vi "Convert Array to IH.vi"(1 "Array":u8[](array[numeric])) -> (0 "IH":T1)   [LabVIEW 2013, in "VRI.lvlib"]
uses:
  VRI.lvlib
  _Type Defs/PhInt IH.ctl
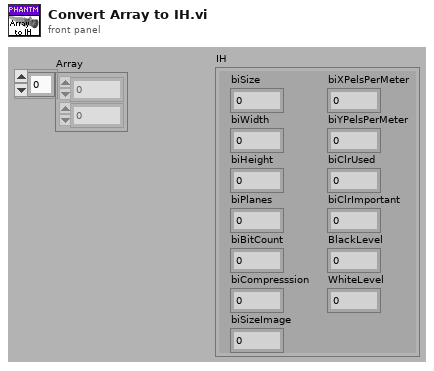
[diagram p1: front panel]
types:
  T1 = typedef "VRI.lvlib/PhInt IH.ctl" = cluster{"biSize":u32, "biWidth":i32, "biHeight":i32, "biPlanes":u16, "biBitCount":u16, "biCompresssion":u32, "biSizeImage":u32, "biXPelsPerMeter":i32, "biYPelsPerMeter":i32, "biClrUsed":u32, "biClrImportant":u32, "BlackLevel":i32, "WhiteLevel":i32}
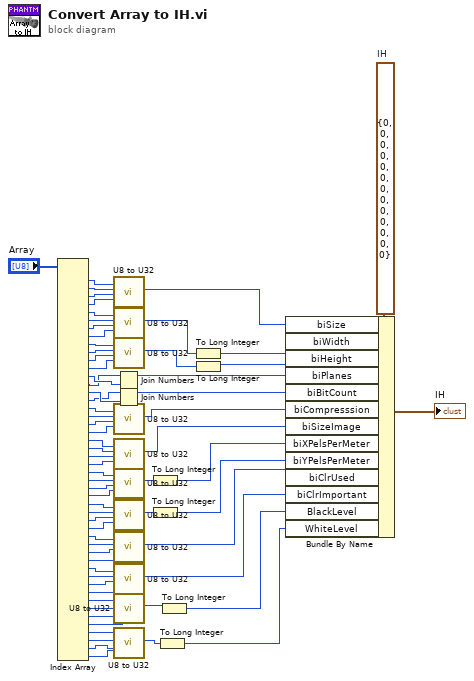
[diagram p0: block diagram]
diagram:
  w14 = T1 {"biSize"=0, "biWidth"=0, "biHeight"=0, "biPlanes"=0, "biBitCount"=0, "biCompresssion"=0, "biSizeImage"=0, "biXPelsPerMeter"=0, "biYPelsPerMeter"=0, "biClrUsed"=0, "biClrImportant"=0, "BlackLevel"=0, "WhiteLevel"=0}  # IH
  n1 = Index Array(array="Array") -> (element #1=w19:u8, element #2=w16:u8, element #3=w18:u8, element #4=w17:u8, element #5=w21:u8, element #6=w22:u8, element #7=w23:u8, element #8=w24:u8, element #9=w25:u8, element #10=w26:u8, element #11=w27:u8, element #12=w28:u8, element #13=w68:u8, element #14=w67:u8, element #15=w70:u8, element #16=w69:u8, element #17=w35:u8, element #18=w36:u8, element #19=w37:u8, element #20=w38:u8, element #21=w39:u8, element #22=w40:u8, element #23=w41:u8, element #24=w42:u8, element #25=w47:u8, element #26=w48:u8, element #27=w49:u8, element #28=w50:u8, element #29=w51:u8, element #30=w52:u8, element #31=w53:u8, element #32=w54:u8, element #33=w56:u8, element #34=w57:u8, element #35=w58:u8, element #36=w59:u8, element #37=w60:u8, element #38=w61:u8, element #39=w62:u8, element #40=w63:u8, element #41=w12:u8, element #42=w11:u8, element #43=w10:u8, element #44=w9:u8, element #45=w8:u8, element #46=w7:u8, element #47=w5:u8, element #48=w6:u8)  [unwired: 48 in]
  n2 = call "U8 to U32.vi"("Byte1"=w19, "Byte2"=w16, "Byte3"=w18, "Byte4"=w17) -> ("U32"=w20:u32)  [unwired: 1 in, 14 out]
  n3 = call "U8 to U32.vi"("Byte1"=w21, "Byte2"=w22, "Byte3"=w23, "Byte4"=w24) -> ("U32"=w29:u32)  [unwired: 1 in, 14 out]
  n4 = call "U8 to U32.vi"("Byte1"=w25, "Byte2"=w26, "Byte3"=w27, "Byte4"=w28) -> ("U32"=w30:u32)  [unwired: 1 in, 14 out]
  n5 = Join Numbers(hi=w67, lo=w68) -> ((hi.lo)=w33:u16)
  n6 = Join Numbers(hi=w69, lo=w70) -> ((hi.lo)=w34:u16)
  n7 = call "U8 to U32.vi"("Byte1"=w35, "Byte2"=w36, "Byte3"=w37, "Byte4"=w38) -> ("U32"=w43:u32)  [unwired: 1 in, 14 out]
  n8 = call "U8 to U32.vi"("Byte1"=w39, "Byte2"=w40, "Byte3"=w41, "Byte4"=w42) -> ("U32"=w44:u32)  [unwired: 1 in, 14 out]
  n9 = call "U8 to U32.vi"("Byte1"=w47, "Byte2"=w48, "Byte3"=w49, "Byte4"=w50) -> ("U32"=w46:u32)  [unwired: 1 in, 14 out]
  n10 = call "U8 to U32.vi"("Byte1"=w51, "Byte2"=w52, "Byte3"=w53, "Byte4"=w54) -> ("U32"=w45:u32)  [unwired: 1 in, 14 out]
  n11 = call "U8 to U32.vi"("Byte1"=w56, "Byte2"=w57, "Byte3"=w58, "Byte4"=w59) -> ("U32"=w64:u32)  [unwired: 1 in, 14 out]
  n12 = call "U8 to U32.vi"("Byte1"=w60, "Byte2"=w61, "Byte3"=w62, "Byte4"=w63) -> ("U32"=w65:u32)  [unwired: 1 in, 14 out]
  n13 = call "U8 to U32.vi"("Byte1"=w12, "Byte2"=w11, "Byte3"=w10, "Byte4"=w9) -> ("U32"=w4:u32)  [unwired: 1 in, 14 out]
  n14 = call "U8 to U32.vi"("Byte1"=w8, "Byte2"=w7, "Byte3"=w5, "Byte4"=w6) -> ("U32"=w2:u32)  [unwired: 1 in, 14 out]
  n15 = To Long Integer(number=w46) -> (32bit integer=w66:i32)
  n16 = To Long Integer(number=w45) -> (32bit integer=w55:i32)
  n17 = To Long Integer(number=w2) -> (32bit integer=w1:i32)
  n18 = To Long Integer(number=w4) -> (32bit integer=w3:i32)
  n19 = To Long Integer(number=w29) -> (32bit integer=w31:i32)
  n20 = To Long Integer(number=w30) -> (32bit integer=w32:i32)
  n21 = Bundle By Name(cluster=w14, "biSize"=w20, "biWidth"=w31, "biHeight"=w32, "biPlanes"=w33, "biBitCount"=w34, "biCompresssion"=w43, "biSizeImage"=w44, "biXPelsPerMeter"=w66, "biYPelsPerMeter"=w55, "biClrUsed"=w64, "biClrImportant"=w65, "BlackLevel"=w3, "WhiteLevel"=w1) -> (→"IH":T1)
